vi "start receiver loop.vi"(8 "error in":errorcluster, 11 "socket reference":T2) -> (0 "error out":errorcluster, 3 "receiver reference":T1)   [LabVIEW 2013, in "lvnano.lvlib"]
uses:
  lvnano.lvlib
  socket reference.ctl
  receive loop reference.ctl
  lvnanomsg.dll
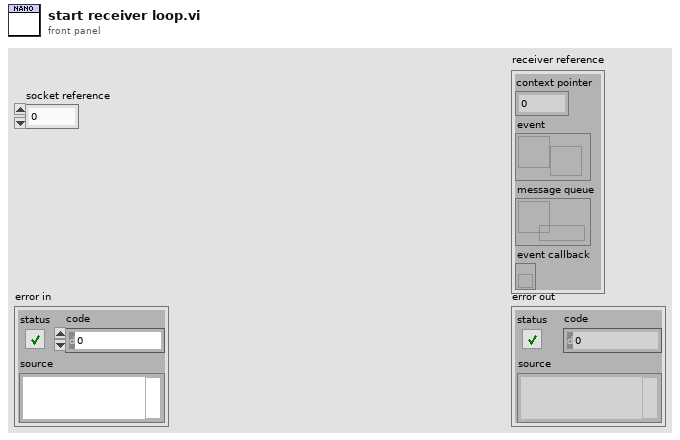
[diagram p1: front panel]
types:
  T1 = typedef "lvnano.lvlib/receive loop reference.ctl" = cluster{"context pointer":i64, "event":refnum<user-event>, "message queue":refnum<queue>, "event callback":refnum<k27>}
  T2 = typedef "lvnano.lvlib/socket reference.ctl" = i64
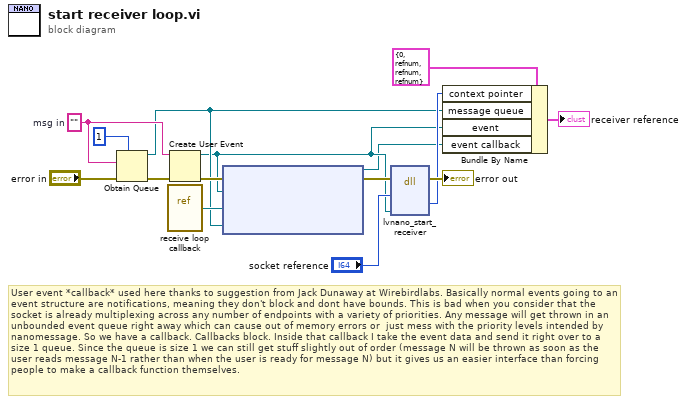
[diagram p0: block diagram]
diagram:
  w14 = ""  # msg in
  # "User event *callback* used here thanks to suggestion from Jack Dunaway at Wirebirdlabs. Basically normal events going to an event structure are notifications, meaning they don't block and dont have bounds. This is bad when you consider that the socket is already multiplexing across any number of endpoints with a variety of priorities. Any message will get thrown in an unbounded event queue right away which can cause out of memory errors or  just mess with the priority levels intended by nanomessage. So we have a callback. Callbacks block. Inside that callback I take the event data and send it right over to a size 1 queue. Since the queue is size 1 we can still get stuff slightly out of order (message N will be thrown as soon as the user reads message N-1 rather than when the user is ready for message N) but it gives us an easier interface than forcing people to make a callback function themselves."
  n1 = Obtain Queue(max queue size (-1, unlimited)=1, element data type=w14, error in (no error)="error in") -> (queue out=w3:refnum<queue>, error out=w15:errorcluster)  [unwired: 2 in, 1 out]
  n2 = vi-ref "receive loop callback.vi"() -> ("vi reference"=w4:refnum<vi>)
  n3 = Create User Event(user event datatype=w14, error in=w15) -> (user event=w2:refnum<user-event>, error out=w7:errorcluster)
  n4 = node(w7, w2, w4, w3) -> (w1:refnum<k27>, w6:errorcluster)  [unwired: 1 in]
  n5 = dll-call lib="C:/Users/Daniel/Documents/nanomsg/lvnano/lvnanomsg.*" fn="lvnano_start_receiver"(error in=w6, "s"="socket reference", "event"=w2) -> (error out=→"error out":errorcluster, "rthread context pointer"=w8:i64)  [unwired: 6 in, 1 out]
  n6 = Bundle By Name(cluster=T1 {"context pointer"=0, "event"=refnum, "message queue"=refnum, "event callback"=refnum} ("receiver reference"), "context pointer"=w8, "message queue"=w3, "event"=w2, "event callback"=w1) -> (→"receiver reference":T1)
